vi "Flatten Message To String.vi"(0 "message":T1, 11 "error in":errorcluster) -> (4 "message string":string, 15 "error out":errorcluster)   [LabVIEW 2015, in "TLB` Template.lvlib" / "AMC.lvlib"]
doc: "TLB Prime - Application Template 1.3.0.24\nNorm Kirchner, NI Systems Engineering - NI\nCopyright (c) 2014, NI"
uses:
  AMC.lvlib
  Message.ctl
  Tools/Keyed Array/KeyedArray.ctl
  Tools/Keyed Array/Tools_KeyedArray.lvlib
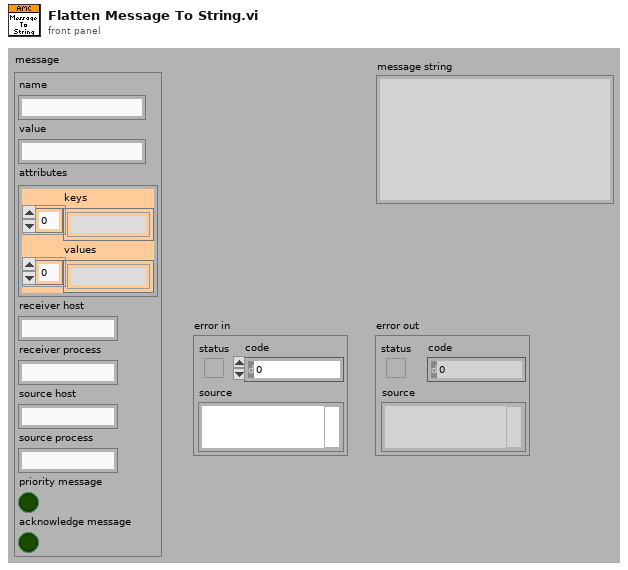
[diagram p1: front panel]
types:
  T1 = typedef "TLB` Template.lvlib/AMC.lvlib/Message.ctl" = cluster{"name":string, "value":string, "attributes":T2, "receiver host":string, "receiver process":string, "source host":string, "source process":string, "priority message":bool, "acknowledge message":bool}
  T2 = typedef "TLB` Template.lvlib/Tools_KeyedArray.lvlib/KeyedArray.ctl" = cluster{"keys":string[], "values":string[]}
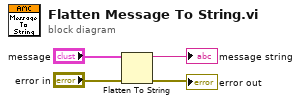
[diagram p0: block diagram]
diagram:
  n1 = Flatten To String(anything="message", error in (no error)="error in") -> (data string=→"message string":string, error out=→"error out":errorcluster)  [unwired: 2 in, 1 out]
